vi "Part 1.vi"(11 "Input":string) -> (3 "Output":i64)   [LabVIEW 2021]
uses:
  <userlib>/_OpenG.lib/string/string.llb/Convert EOLs (String)__ogtk.vi
panel:
  in  "Tab Control":enum32{"Graph", "Intensity"}(tab)
  out "Lines":cluster{cluster{i32, i32}[]}[](graph)
  out "Grid":i64[][](graph)
  out "min y":i32
  out "max y":i32
  out "min x":i32
  out "max x":i32
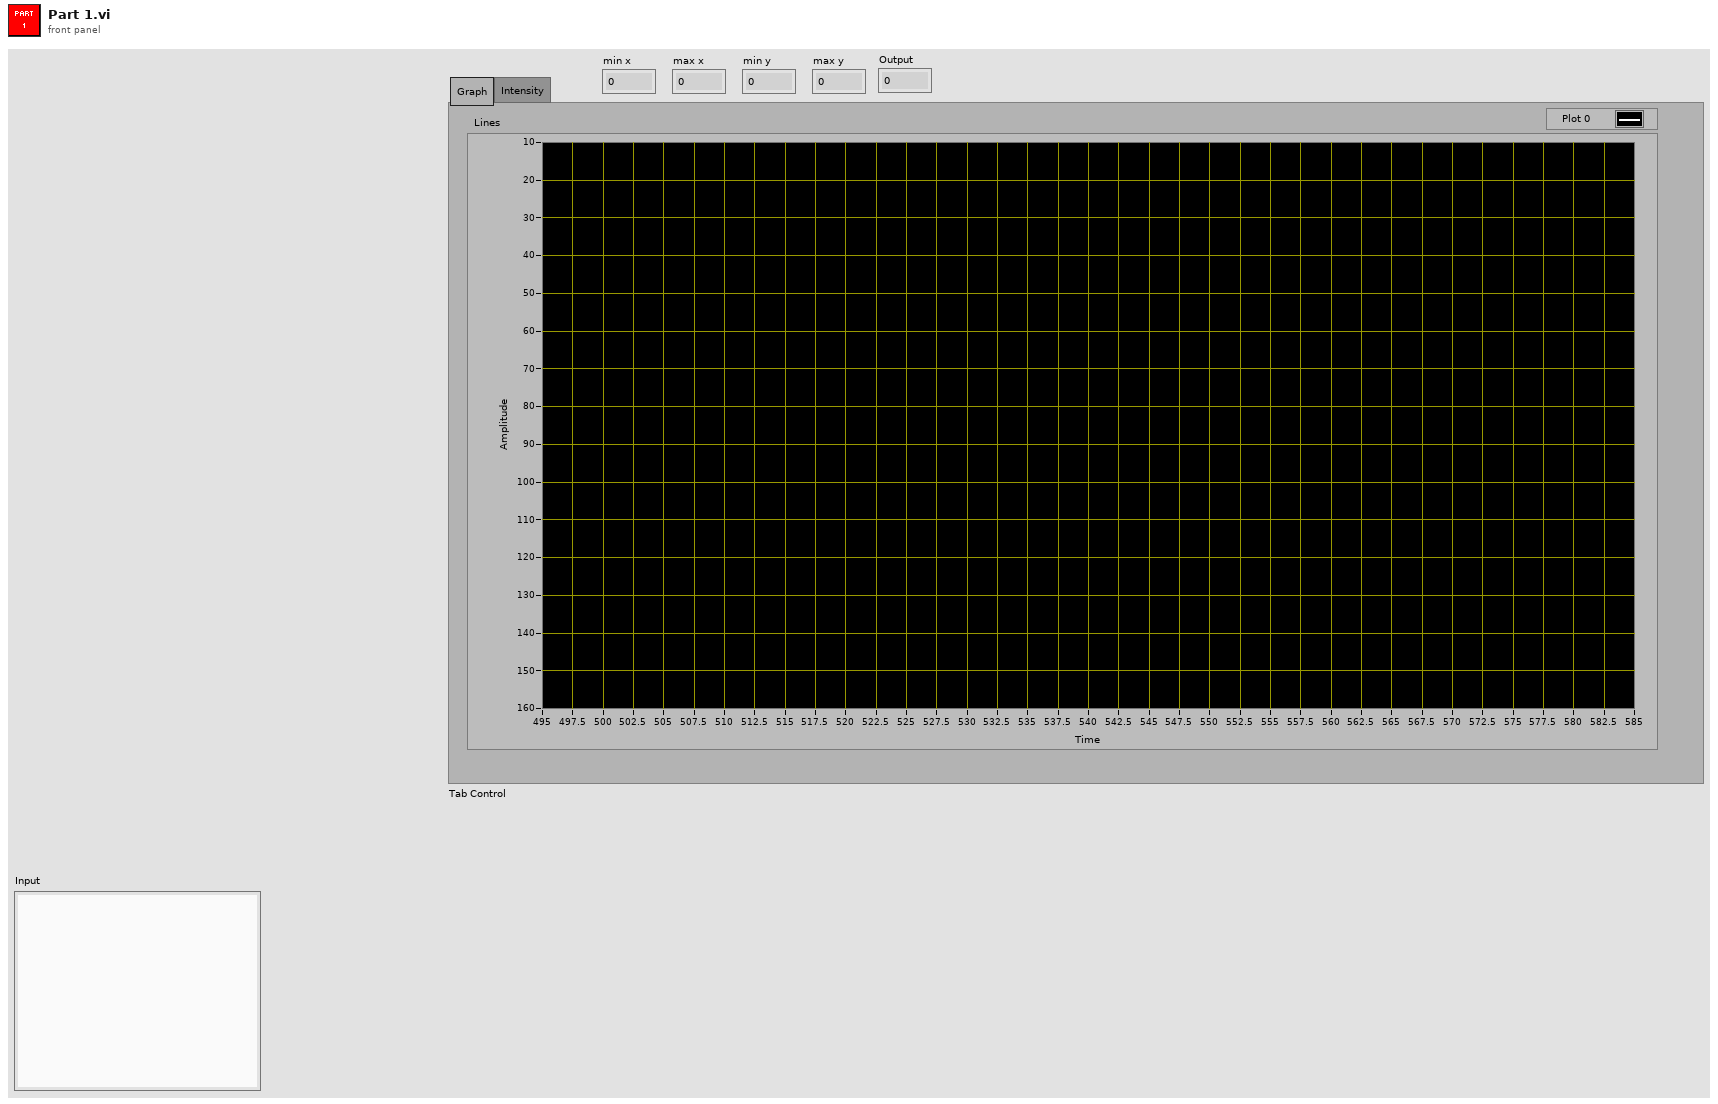
[diagram p1: front panel]
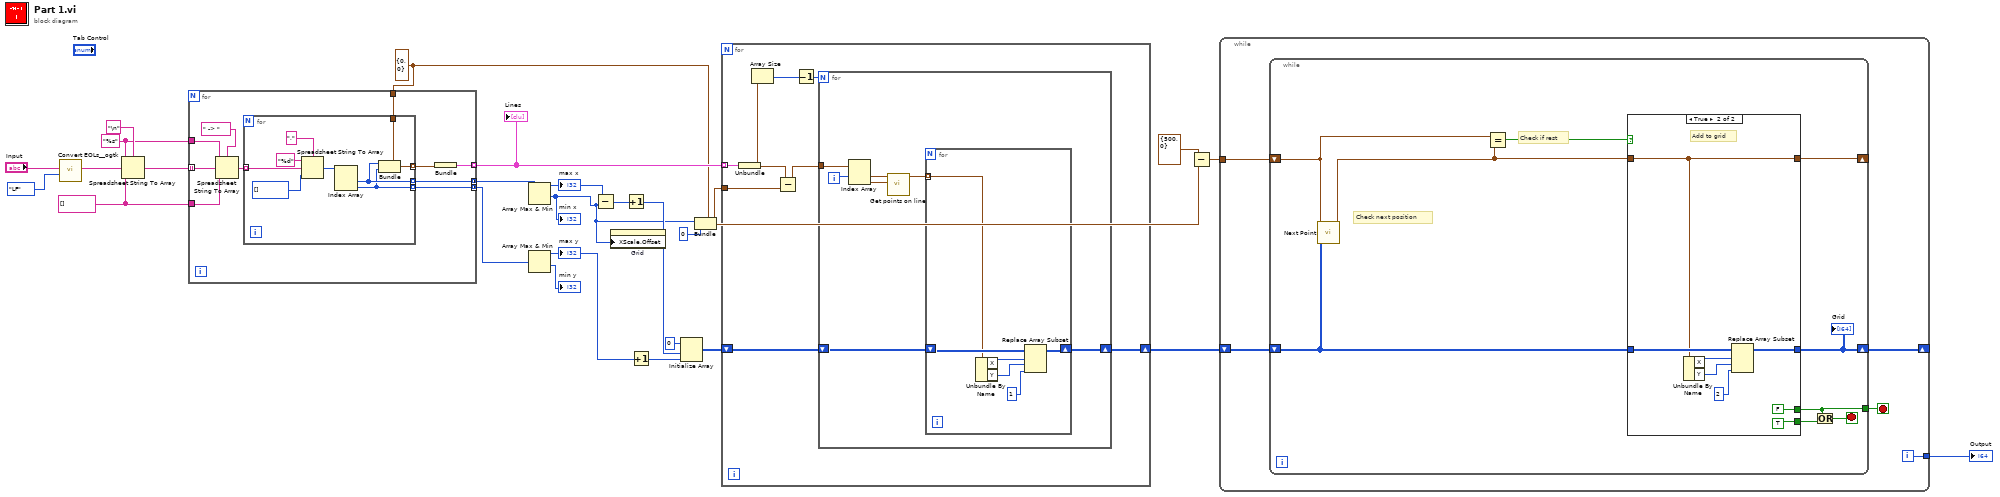
[diagram p0: block diagram]
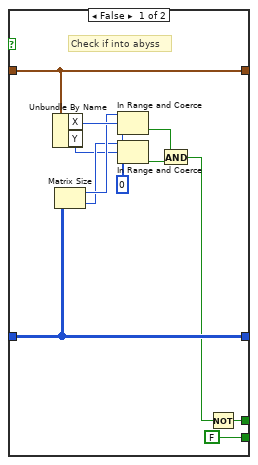
[diagram p2: hidden frame]
diagram:
  w2 = cluster{"X":i32, "Y":i32} {"X"=0, "Y"=0} ("cluster")
  w20 = string[] []
  w21 = "%s"
  n1 = call-poly <userlib>:"Convert EOLs__ogtk.vi"("Convert to:"=enum16{"CR", "LF", "CRLF"}."LF", "String in"="Input") -> ("String out"=w24:string)  [unwired: 9 in]
  n2 = Spreadsheet String To Array(delimiter (Tab)="\n", format string=w21, spreadsheet string=w24, array type (2D Dbl)=w20) -> (array=w22:string[])
  n3 = for {
    tunnel: w22 -> [w34] mode=indexing
    tunnel: w21 -> [w36]
    tunnel: w20 -> [w35]
    tunnel: [w31] -> w17 mode=concatenating
    tunnel: [w30] -> w18 mode=concatenating
    tunnel: [w28] -> w12 mode=indexing
    tunnel: w2 -> [w27]
    n4 = Spreadsheet String To Array(delimiter (Tab)=" -> ", format string=w36, spreadsheet string=w34, array type (2D Dbl)=w35) -> (array=w32:string[])
    n5 = for {
      tunnel: w32 -> [w45] mode=indexing
      tunnel: [w40] -> w31 mode=indexing
      tunnel: [w39] -> w30 mode=indexing
      tunnel: [w38] -> w29 mode=indexing
      tunnel: w27 -> [w37]
      n6 = Spreadsheet String To Array(delimiter (Tab)=",", format string="%d", spreadsheet string=w45, array type (2D Dbl)=i32[] []) -> (array=w41:i32[])
      n7 = Index Array(array=w41) -> (element #1=w40:i32, element #2=w39:i32)  [unwired: 2 in]
      n8 = Bundle(cluster=w37, "X"=w40, "Y"=w39) -> (w38:cluster{"X":i32, "Y":i32})
    }
    n9 = Bundle(w29) -> (w28:cluster{cluster{"X":i32, "Y":i32}[]})  [unwired: 1 in]
  }
  "Lines" <- w12
  n10 = Array Max & Min(array=w17) -> (max value=w16:i32, min value=w9:i32)  [unwired: 2 out]
  "max x" <- w16
  "min x" <- w9
  n11 = Array Max & Min(array=w18) -> (max value=w11:i32, min value=→"min y":i32)  [unwired: 2 out]
  "max y" <- w11
  n12 = Subtract(x=w16, y=w9) -> (x-y=w15:i32)
  n13 = property on="Grid" class="IntGraph (strict)"("XScale.Offset"=w9) -> ()  [unwired: 2 in, 2 out]
  n14 = Increment(x=w15) -> (x+1=w10:i32)
  n15 = Increment(x=w11) -> (x+1=w8:i32)
  n16 = Initialize Array(i64 0 ("element"), w10, w8) -> (w13:i64[][])
  n17 = Bundle(cluster=w2, "X"=w9, "Y"=0 ("min x")) -> (w4:cluster{"X":i32, "Y":i32})
  n18 = for {
    shift-right: [w49] -> w7
    shift-left: w13 -> [w50]
    tunnel: w12 -> [w53] mode=indexing
    tunnel: w4 -> [w46]
    n19 = Unbundle(w53) -> (w48:cluster{"X":i32, "Y":i32}[])
    n20 = Array Size(array=w48) -> (size(s)=w52:i32)
    n21 = Subtract(x=w48, y=w46) -> (x-y=w47:cluster{"X":i32, "Y":i32}[])
    n22 = Decrement(x=w52) -> (x-1=w51:i32)
    n23 = for {
      N: w51 -> [_]
      tunnel: w47 -> [w60]
      shift-right: [w54] -> w49
      shift-left: w50 -> [w55]
      i -> [w59]
      n24 = Index Array(array=w60, index #1=w59) -> (element #1=w58:cluster{"X":i32, "Y":i32}, element #2=w57:cluster{"X":i32, "Y":i32})  [unwired: 1 in]
      n25 = call "Get points on line.vi"("Stop"=w57, "Start"=w58) -> ("Line"=w56:cluster{"X":i32, "Y":i32}[])  [unwired: 9 in]
      n26 = for {
        tunnel: w56 -> [w64] mode=indexing
        shift-right: [w65] -> w54
        shift-left: w55 -> [w66]
        n27 = Unbundle By Name(w64) -> ("X"=w63:i32, "Y"=w62:i32)
        n28 = Replace Array Subset(array=w66, new element=i64 1 ("new element/subarray"), index (row)=w63, index (col)=w62) -> (w65:i64[][])
      }
    }
  }
  n29 = Subtract(x=cluster{"X":i32, "Y":i32} {"X"=500, "Y"=0} ("Rest"), y=w4) -> (x-y=w3:cluster{"X":i32, "Y":i32})
  n30 = while {
    shift-right: [w70] -> _
    shift-left: w7 -> [w71]
    tunnel: [w69] -> w1
    tunnel: w3 -> [w68]
    i -> [w69]
    stop <- w67 stop-if-true
    n31 = while {
      shift-right: [w79] -> w70
      shift-left: w71 -> [w74]
      shift-right: [w78] -> _
      shift-left: w68 -> [w72]
      tunnel: [w75] -> w67
      stop <- w80 stop-if-true
      # "Check if rest"
      # "Check next position"
      n32 = call "Next Point.vi"("Grid In"=w74, "Point"=w72) -> ("Point out"=w73:cluster{"X":i32, "Y":i32})  [unwired: 9 in]
      n33 = Equal?(x=w72, y=w73) -> (x = y?=w77:bool)
      n34 = case shown="True" w77 {
        tunnel: [w81 FALSE] -> w75
        tunnel: w73 -> [w91 w93]
        tunnel: w74 -> [w90 w95]
        tunnel: [w90 w94] -> w79
        tunnel: [w91 w93] -> w78
        tunnel: [FALSE TRUE] -> w76
        frame False {
          w85 = 0 ("lower limit")
          # "Check if into abyss"
          n35 = Unbundle By Name(w91) -> ("X"=w89:i32, "Y"=w86:i32)
          n36 = Matrix Size(0:w90) -> (1:w88:i32, 2:w87:i32)
          n37 = In Range and Coerce(upper limit=w88, x=w89, lower limit=w85) -> (In Range?=w83:bool)  [unwired: 1 out]
          n38 = In Range and Coerce(upper limit=w87, x=w86, lower limit=w85) -> (In Range?=w84:bool)  [unwired: 1 out]
          n39 = And(x=w83, y=w84) -> (x .and. y?=w82:bool)
          n40 = Not(x=w82) -> (.not. x?=w81:bool)
        }
        frame True {
          # "Add to grid"
          n41 = Unbundle By Name(w93) -> ("X"=w98:i32, "Y"=w97:i32)
          n42 = Replace Array Subset(array=w95, new element=i64 2 ("new element/subarray"), index (row)=w98, index (col)=w97) -> (w94:i64[][])
        }
      }
      "Grid" <- w79
      n43 = Or(x=w75, y=w76) -> (x .or. y?=w80:bool)
    }
  }
  "Output" <- w1
